vi "Get Base Protocol.vi"(8 "error in (no error)":errorcluster, 11 "Protocol Parent in":refnum<class "Protocol Parent.lvclass">) -> (0 "error out":errorcluster, 2 "Protocol out":T1, 3 "Protocol Parent out":refnum<class "Protocol Parent.lvclass">)   [LabVIEW 2019, in "Protocols.lvlib" / "Protocol Parent.lvclass"]
uses:
  Protocol Parent.lvclass
  Types/Base Protocol Type.ctl
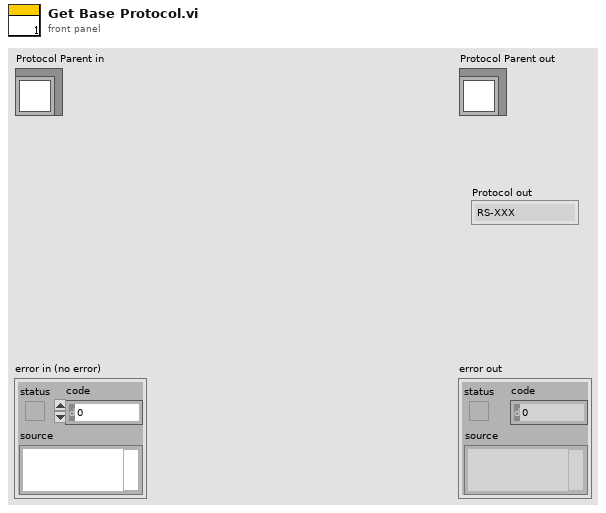
[diagram p1: front panel]
types:
  T1 = typedef "Protocols.lvlib/Protocol Parent.lvclass/Base Protocol Type.ctl" = enum16{"RS-XXX", "VISA", "TCPIP", "UDP", "GPIB ConvBox"}
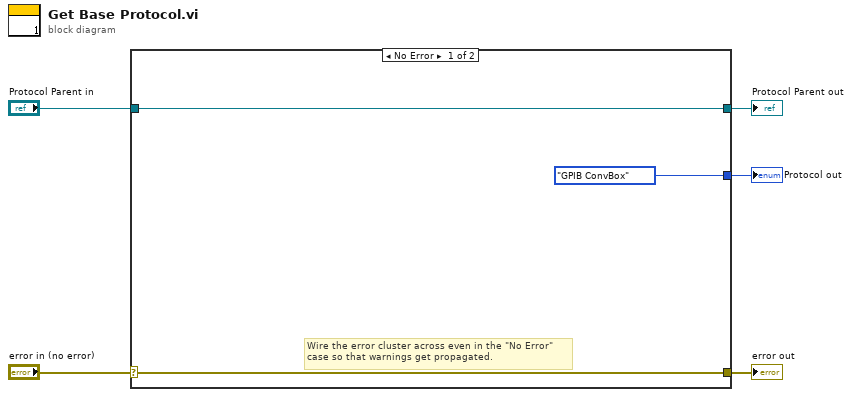
[diagram p0: block diagram]
diagram:
  n1 = case shown="No Error" "error in (no error)" {
    selector: "error in (no error)" -> [w7 w10]
    tunnel: [w7 w10] -> w4
    tunnel: [w8 w9] -> w2
    tunnel: "Protocol Parent in" -> [w8 w9]
    tunnel: [Base_Protocol_Type."GPIB ConvBox" ("Protocol out") _] -> w1
    frame No Error {
      # "Wire the error cluster across even in the \"No Error\"\ncase so that warnings get propagated."
    }
    frame Error {
    }
  }
  "error out" <- w4
  "Protocol Parent out" <- w2
  "Protocol out" <- w1
